vi "PE Get Status Str.vi"(8 "error in (no error)":errorcluster, 11 "code":i32) -> (0 "error out":errorcluster, 3 "function return":string)   [LabVIEW 2011, in "libPhyspec.lvlib"]
doc: "PHYSPEC_API const char* PE_GetStatusStr(PE_STATUS code);"
uses:
  libPhyspec.lvlib
  libPhyspec.dll
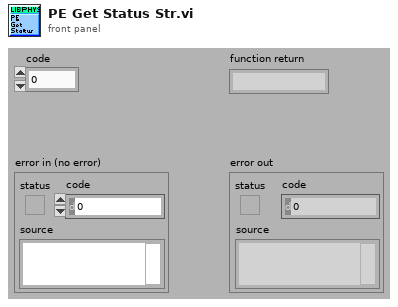
[diagram p1: front panel]
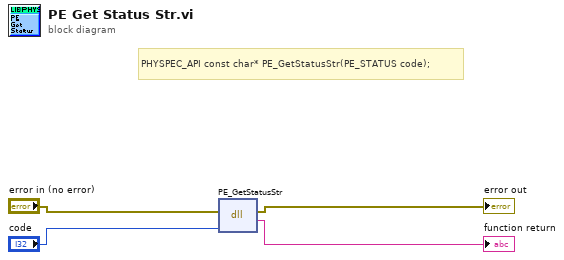
[diagram p0: block diagram]
diagram:
  # "PHYSPEC_API const char* PE_GetStatusStr(PE_STATUS code);"
  n1 = dll-call lib="D:/users/nicolas/PHySpec-SDK-1.0.0/Labview-example/libPhyspec/libPhyspec.*" fn="PE_GetStatusStr"(error in="error in (no error)", "code"="code") -> (error out=→"error out":errorcluster, →"function return":string)  [unwired: 3 in, 1 out]
